vi "短日期时间转长日期格式.vi"(10 "table输入":string(combo), 11 "data":string[][](table)) -> (3 "输出数组":string[][](array[string]))   [LabVIEW 2016]
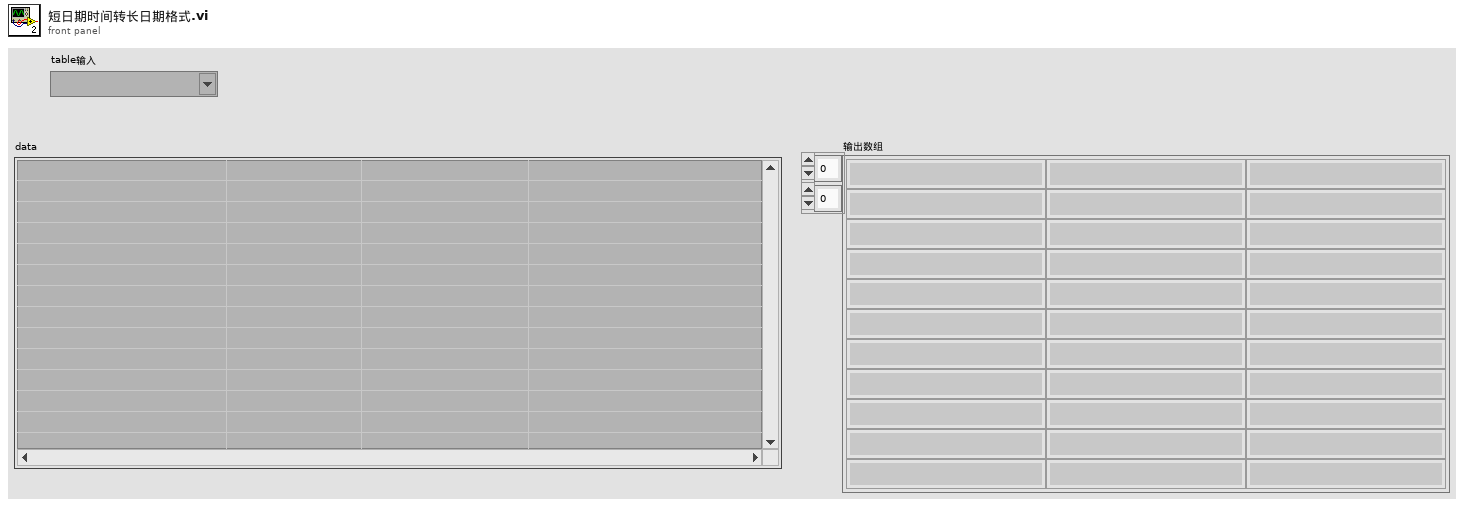
[diagram p1: front panel]
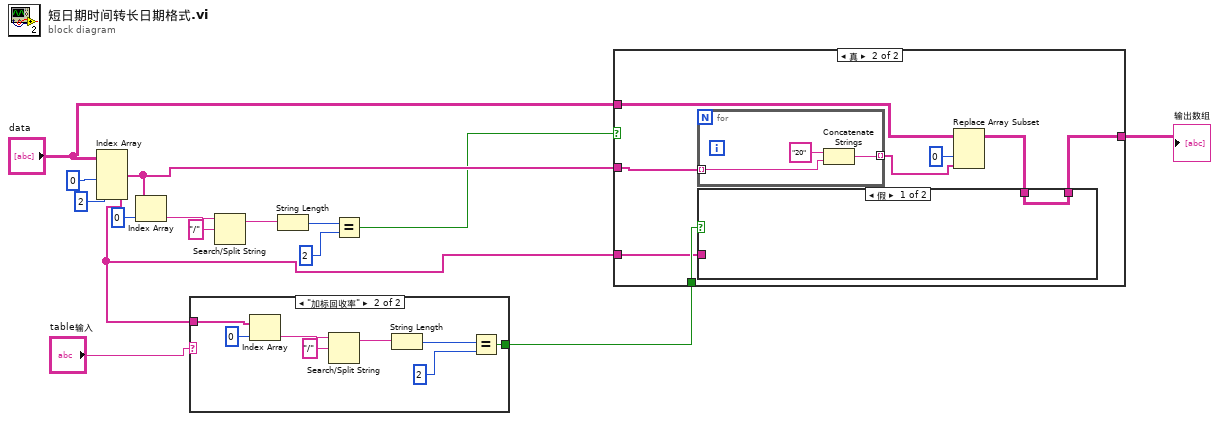
[diagram p0: block diagram]
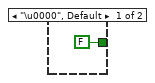
[diagram p2: hidden frame]
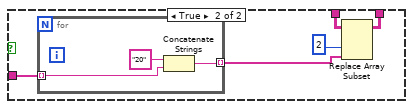
[diagram p4: hidden frame]
diagram:
  n1 = Index Array(array="data", index (col) #1=0 ("禁用的索引 (列)"), index (col) #2=2 ("索引 (列)")) -> (element #1=w12:string[], element #2=w2:string[])  [unwired: 2 in]
  n2 = Index Array(array=w12, index=0 ("索引")) -> (element=w10:string)
  n3 = case shown="\"加标回收率\"" "table输入" {
    tunnel: [FALSE w18] -> w3
    tunnel: w2 -> [_ w17]
    frame "\u0000", Default {
    }
    frame "加标回收率" {
      n4 = Index Array(array=w17, index=0 ("索引")) -> (element=w20:string)
      n5 = Search/Split String(string=w20, search string/char (-)="/" ("搜索字符串/字符(-)")) -> (substring before match=w22:string)  [unwired: 1 in, 2 out]
      n6 = String Length(string=w22) -> (length=w23:i32)
      n7 = Equal?(x=w23, y=2) -> (x = y?=w18:bool)
    }
  }
  n8 = Search/Split String(string=w10, search string/char (-)="/" ("搜索字符串/字符(-)")) -> (substring before match=w8:string)  [unwired: 1 in, 2 out]
  n9 = String Length(string=w8) -> (length=w7:i32)
  n10 = Equal?(x=w7, y=2) -> (x = y?=w5:bool)
  n11 = case shown="真" w5 {
    tunnel: w12 -> [_ w33]
    tunnel: "data" -> [w25 w32]
    tunnel: [w25 w28] -> w13
    tunnel: w3 -> [_ w27]
    tunnel: w2 -> [_ w26]
    frame False {
    }
    frame True {
      n12 = for {
        tunnel: w33 -> [w45] mode=indexing
        tunnel: [w43] -> w30 mode=indexing
        n13 = Concatenate Strings("20" ("字符串"), w45) -> (w43:string)
      }
      n14 = Replace Array Subset(array=w32, new element=w30, index (col)=0 ("禁用的索引 (列)")) -> (w29:string[][])  [unwired: 1 in]
      n15 = case shown="假" w27 {
        tunnel: w29 -> [w34 w38]
        tunnel: [w34 w37] -> w28
        tunnel: w26 -> [_ w35]
        frame False {
        }
        frame True {
          n16 = for {
            tunnel: [w41] -> w36 mode=indexing
            tunnel: w35 -> [w40] mode=indexing
            n17 = Concatenate Strings("20" ("字符串"), w40) -> (w41:string)
          }
          n18 = Replace Array Subset(array=w38, new element=w36, index (col)=2 ("索引 (列)")) -> (w37:string[][])  [unwired: 1 in]
        }
      }
    }
  }
  "输出数组" <- w13
